vi "奇异点删除.vi"(7 "原始角点坐标":cluster{"X":sgl, "Y":sgl}[](array[cluster]), 9 "Image In":T1) -> (1 "原始角点坐标 2":cluster{"X":sgl, "Y":sgl}[](array[cluster]), 3 "角点图":T1(plugin-control))   [LabVIEW 2018]
uses:
  <vilib>/vision/Image Controls.llb/IMAQ Image.ctl
panel:
  in  "刷新按钮":bool
  in  "快进按钮":bool
  in  "操作类型":bool
  in  "y":i32
  in  "停止角点删除":bool
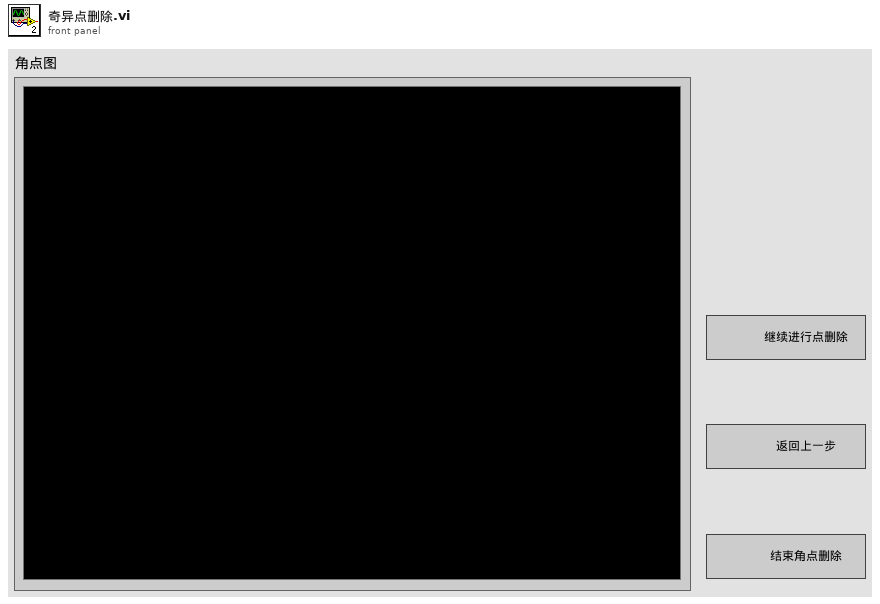
[diagram p1: front panel]
types:
  T1 = typedef "IMAQ Image.ctl" = refnum<image>
  T2 = typedef "IMAQ Rectangle" = cluster{"Left":i32, "Top":i32, "Right":i32, "Bottom":i32, "Rotation":dbl}
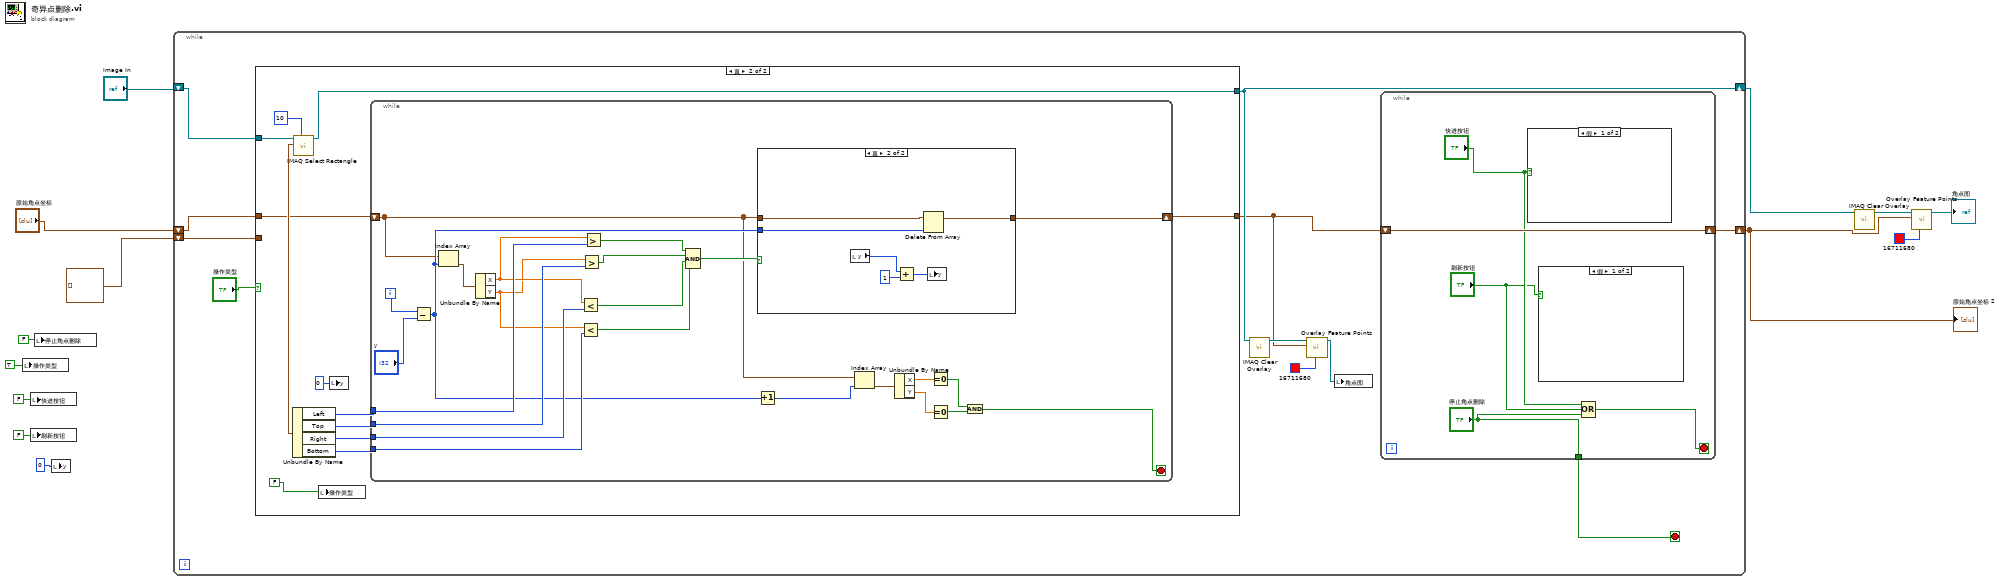
[diagram p0: block diagram]
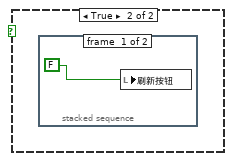
[diagram p2: hidden frame]
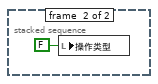
[diagram p3: hidden frame]
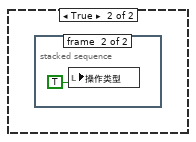
[diagram p4: hidden frame]
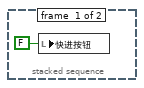
[diagram p5: hidden frame]
diagram:
  n1 = local write "操作类型"(TRUE) -> ()
  n2 = local write "快进按钮"(FALSE ("快进按钮")) -> ()
  n3 = local write "刷新按钮"(FALSE ("刷新按钮")) -> ()
  n4 = local write "停止角点删除"(FALSE ("停止角点删除")) -> ()
  n5 = local write "y"(0 ("y")) -> ()
  n6 = while {
    shift-right: [w17] -> w10
    shift-left: "原始角点坐标" -> [w15]
    shift-left: cluster{"X":sgl, "Y":sgl}[] [] ("原始角点坐标") -> [w16]
    shift-right: [w21] -> w8
    shift-left: "Image In" -> [w19]
    stop <- w14 stop-if-true
    n7 = case shown="真" "操作类型" {
      tunnel: w15 -> [_ w43]
      tunnel: w19 -> [w35 w41]
      tunnel: [w34 w40] -> w18
      tunnel: [w35 w39] -> w21
      tunnel: w16 -> [w34 _]
      frame False {
      }
      frame True {
        n8 = call "IMAQ Select Rectangle"("Window Number (0...15)"=10, "Image In"=w41) -> ("Rectangle"=w47:T2, "Image Out (duplicate)"=w39:T1)  [unwired: 6 in, 2 out]
        n9 = Unbundle By Name(w47) -> ("Left"=w46:i32, "Top"=w42:i32, "Right"=w44:i32, "Bottom"=w45:i32)
        n10 = local write "操作类型"(FALSE) -> ()
        n11 = local write "y"(0 ("y")) -> ()
        n12 = while {
          tunnel: w42 -> [w70]
          tunnel: w46 -> [w69]
          tunnel: w45 -> [w58]
          tunnel: w44 -> [w61]
          shift-right: [w54] -> w40
          shift-left: w43 -> [w52]
          i -> [w63]
          stop <- w55 stop-if-true
          n13 = Subtract(x=w63, y="y") -> (x-y=w53:i32)
          n14 = Index Array(array=w52, index=w53) -> (element=w71:cluster{"X":sgl, "Y":sgl})
          n15 = Unbundle By Name(w71) -> ("X"=w60:sgl, "Y"=w59:sgl)
          n16 = Less?(x=w60, y=w61) -> (x < y?=w66:bool)
          n17 = Less?(x=w59, y=w58) -> (x < y?=w65:bool)
          n18 = Greater?(x=w59, y=w70) -> (0:w67:bool)
          n19 = Greater?(x=w60, y=w69) -> (0:w64:bool)
          n20 = Compound Arithmetic op=AND(w64, w67, w66, w65) -> (w68:bool)
          n21 = case shown="真" w68 {
            tunnel: w52 -> [w72 w78]
            tunnel: [w72 w77] -> w54
            tunnel: w53 -> [_ w73]
            frame False {
            }
            frame True {
              n22 = local read "y"() -> (w76:i32)
              n23 = Add(x=w76, y=1) -> (x+y=w74:i32)
              n24 = Delete From Array(array=w78, index=w73) -> (array with subset deleted=w77:cluster{"X":sgl, "Y":sgl}[])  [unwired: 1 in, 1 out]
              n25 = local write "y"(w74) -> ()
            }
          }
          n26 = Increment(x=w53) -> (x+1=w51:i32)
          n27 = Index Array(array=w52, index=w51) -> (element=w50:cluster{"X":sgl, "Y":sgl})
          n28 = Unbundle By Name(w50) -> ("X"=w49:sgl, "Y"=w48:sgl)
          n29 = Equal To 0?(x=w49) -> (x = 0?=w57:bool)
          n30 = Equal To 0?(x=w48) -> (x = 0?=w56:bool)
          n31 = And(x=w57, y=w56) -> (x .and. y?=w55:bool)
        }
      }
    }
    n32 = call "IMAQ Clear Overlay"("Image"=w21) -> ("Image Out"=w24:T1)  [unwired: 9 in, 1 out]
    n33 = call "Overlay Feature Points.vi"("Color"=u32 16711680, "Feature Points"=w18, "Image"=w24) -> ("Image Out"=w20:T1)  [unwired: 7 in, 1 out]
    n34 = local write "角点图"(w20) -> ()
    n35 = while {
      tunnel: ["停止角点删除"] -> w14
      shift-right: [w29] -> w17
      shift-left: w18 -> [w29]
      stop <- w26 stop-if-true
      n36 = case shown="假" "快进按钮" {
        frame False {
        }
        frame True {
          n37 = stacked-sequence {
            frame #0 {
              n38 = local write "快进按钮"(FALSE ("快进按钮")) -> ()
            }
            frame #1 {
              n39 = local write "操作类型"(TRUE) -> ()
            }
          }
        }
      }
      n40 = case shown="假" "刷新按钮" {
        frame False {
        }
        frame True {
          n41 = stacked-sequence {
            frame #0 {
              n42 = local write "刷新按钮"(FALSE) -> ()
            }
            frame #1 {
              n43 = local write "操作类型"(FALSE ("操作类型")) -> ()
            }
          }
        }
      }
      n44 = Compound Arithmetic op=OR("快进按钮", "刷新按钮", "停止角点删除") -> (w26:bool)
    }
  }
  "原始角点坐标 2" <- w10
  n45 = call "IMAQ Clear Overlay"("Image"=w8) -> ("Image Out"=w11:T1)  [unwired: 9 in, 1 out]
  n46 = call "Overlay Feature Points.vi"("Color"=u32 16711680, "Feature Points"=w10, "Image"=w11) -> ("Image Out"=→"角点图":T1)  [unwired: 7 in, 1 out]
